vi "Pad Base64URL for decode.vi"(1 "String in":string) -> (0 "String out":string)   [LabVIEW 2017, in "JSONWebToken.lvclass"]
uses:
  JSONWebToken.lvclass
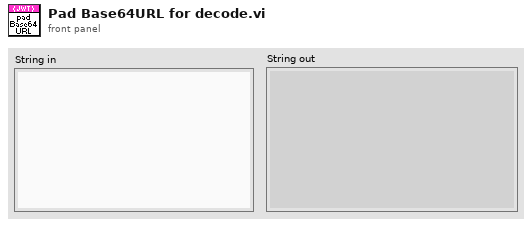
[diagram p1: front panel]
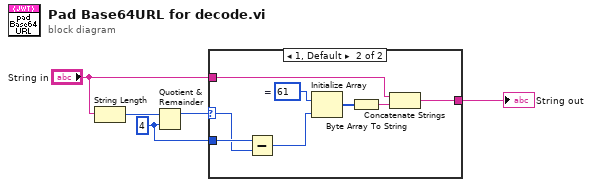
[diagram p0: block diagram]
diagram:
  w1 = 4 ("y")
  n1 = String Length(string="String in") -> (length=w3:i32)
  n2 = Quotient & Remainder(x=w3, y=w1) -> (x-y*floor(x/y)=w2:i32)  [unwired: 1 out]
  n3 = case shown="1, Default" w2 {
    selector: w2 -> [_ w8]
    tunnel: "String in" -> [w6 w13]
    tunnel: [w6 w12] -> w4
    tunnel: w1 -> [_ w9]
    frame 0 {
    }
    frame 1, Default {
      w10 = u8 61  # =
      n4 = Subtract(x=w9, y=w8) -> (x-y=w7:i32)
      n5 = Initialize Array(w10, w7) -> (w11:u8[])
      n6 = Byte Array To String(unsigned byte array=w11) -> (string=w14:string)
      n7 = Concatenate Strings(w13, w14) -> (w12:string)
    }
  }
  "String out" <- w4
